vi "PickingControl.vi"(10 "PickingNumber":string, 11 "Machine":string) -> (0 "error out":errorcluster, 1 "Result":string, 2 "StatusURL":string, 3 "controlURL":string, 4 "DupResult":string)   [LabVIEW 2020]
uses:
  <vilib>/Utility/config.llb/Read Key (String).vi
  <vilib>/Utility/config.llb/NI_LVConfig.lvlib
panel:
  out "Status":bool
  in  "STOP":bool
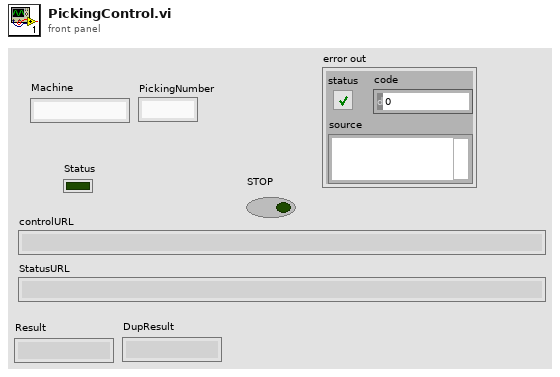
[diagram p1: front panel]
types:
  T1 = typedef "NI_LVConfig.lvlib/Config Data RefNum.ctl" = refnum<k1>
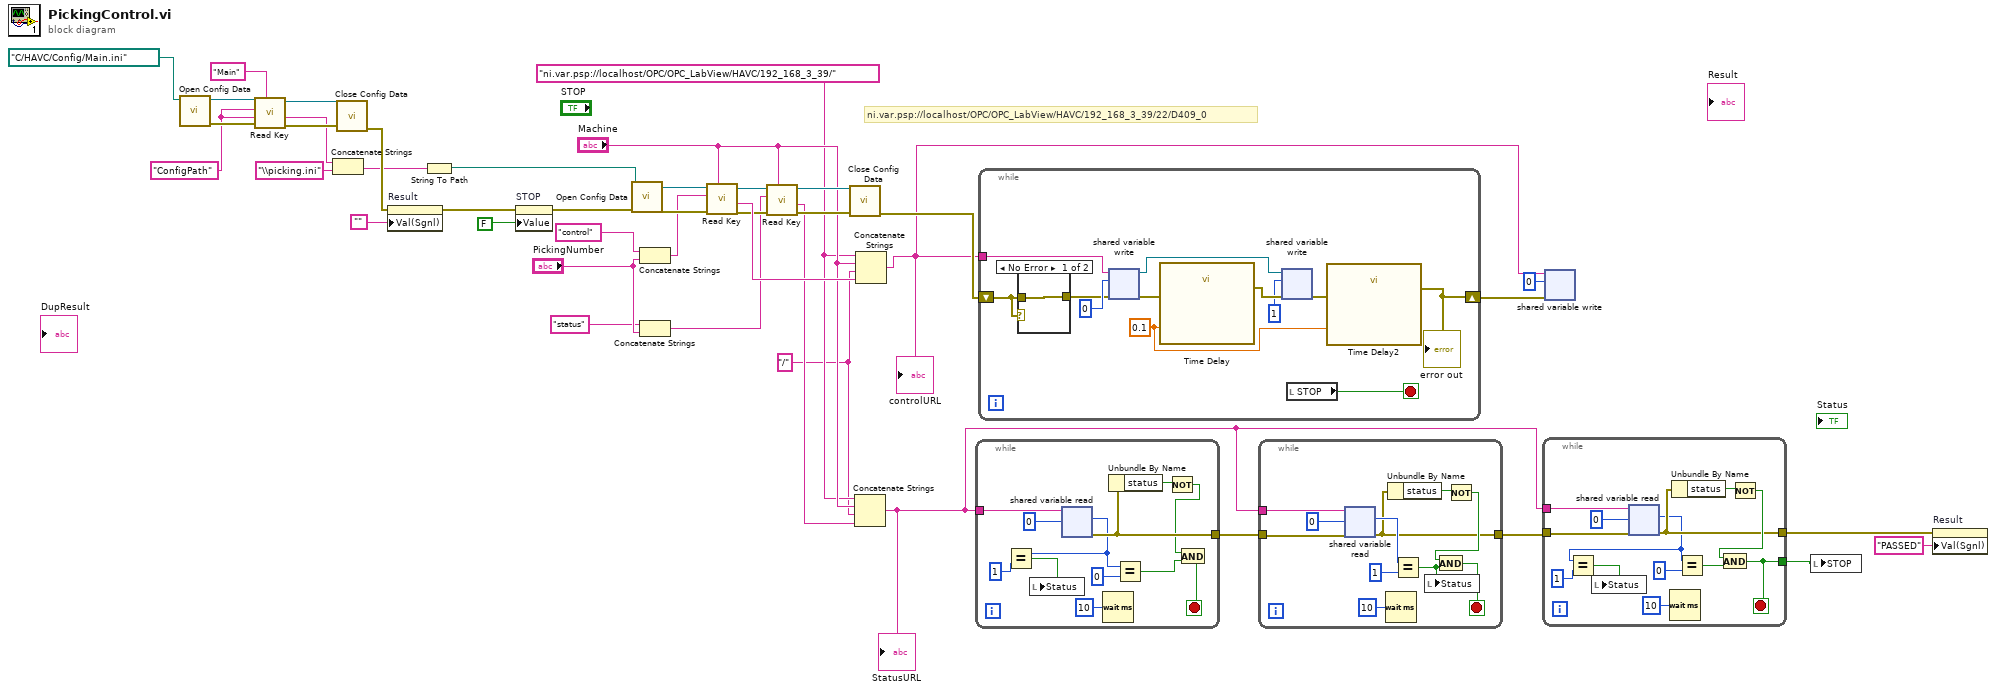
[diagram p0: block diagram]
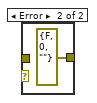
[diagram p2: hidden frame]
diagram:
  w5 = "ConfigPath" ("key")
  w22 = "/" ("string")
  w28 = "ni.var.psp://localhost/OPC/OPC_LabView/HAVC/192_168_3_39/" ("string")
  # "ni.var.psp://localhost/OPC/OPC_LabView/HAVC/192_168_3_39/22/D409_0"
  n1 = call <vilib>:"Open Config Data.vi"("configuration file path"=path "C:/HAVC/Config/Main.ini") -> ("error out"=w11:errorcluster, "refnum"=w10:T1)  [unwired: 8 in, 1 out]
  n2 = call-poly <vilib>:"Read Key.vi"("section"="Main", "error in (no error)"=w11, "default value"=w5, "key"=w5, "refnum"=w10) -> ("error out"=w8:errorcluster, "value"=w4:string, "refnum out"=w9:T1)  [unwired: 3 in, 1 out]
  n3 = Concatenate Strings(w4, "\\picking.ini" ("string")) -> (w2:string)
  n4 = call <vilib>:"Close Config Data.vi"("error in (no error)"=w8, "refnum"=w9) -> ("error out"=w7:errorcluster)  [unwired: 8 in, 1 out]
  n5 = property on="Result" class="Str"(error in=w7, "Val(Sgnl)"="") -> (error out=w14:errorcluster)  [unwired: 1 in, 1 out]
  n6 = String To Path(string=w2) -> (path=w1:path)
  n7 = property on="STOP" class="Bool (strict)"(error in=w14, "Value"=FALSE ("STOP")) -> (error out=w20:errorcluster)  [unwired: 1 in, 1 out]
  n8 = call <vilib>:"Open Config Data.vi"("error in (no error)"=w20, "configuration file path"=w1) -> ("error out"=w42:errorcluster, "refnum"=w41:T1)  [unwired: 7 in, 1 out]
  n9 = Concatenate Strings("control", "PickingNumber") -> (w39:string)
  n10 = Concatenate Strings("status" ("string"), "PickingNumber") -> (w30:string)
  n11 = call-poly <vilib>:"Read Key.vi"("section"="Machine", "error in (no error)"=w42, "key"=w39, "refnum"=w41) -> ("error out"=w34:errorcluster, "value"=w38:string, "refnum out"=w33:T1)  [unwired: 4 in, 1 out]
  n12 = call-poly <vilib>:"Read Key.vi"("section"="Machine", "error in (no error)"=w34, "key"=w30, "refnum"=w33) -> ("error out"=w31:errorcluster, "value"=w23:string, "refnum out"=w32:T1)  [unwired: 4 in, 1 out]
  n13 = call <vilib>:"Close Config Data.vi"("error in (no error)"=w31, "refnum"=w32) -> ("error out"=w37:errorcluster)  [unwired: 8 in, 1 out]
  n14 = Concatenate Strings(w28, "Machine", w22, w23) -> (w25:string)
  "StatusURL" <- w25
  n15 = Concatenate Strings(w28, "Machine", w22, w38) -> (w18:string)
  "controlURL" <- w18
  n16 = while {
    tunnel: w25 -> [w53]
    tunnel: [w49] -> w27
    stop <- w50 stop-if-true
    n17 = shared-variable-read(w53, 0) -> (w49:errorcluster, w45:i32)  [unwired: 1 in, 2 out]
    n18 = Equal?(x=w45, y=1) -> (x = y?=w43:bool)
    n19 = local write "Status"(w43) -> ()
    n20 = Wait (ms)(milliseconds to wait=u32 10) -> ()  [unwired: 1 out]
    n21 = Unbundle By Name(w49) -> ("status"=w48:bool)
    n22 = Equal?(x=w45, y=0) -> (x = y?=w46:bool)
    n23 = Not(x=w48) -> (.not. x?=w47:bool)
    n24 = And(x=w47, y=w46) -> (x .and. y?=w50:bool)
  }
  n25 = while {
    shift-right: [w57] -> w19
    shift-left: w37 -> [w61]
    tunnel: w18 -> [w59]
    stop <- w55 stop-if-true
    w56 = 0.1 ("Delay Time (s)")
    n26 = case shown="No Error" w61 {
      tunnel: w61 -> [w67 _]
      tunnel: [w67 errorcluster {"status"=FALSE, "code"=0, "source"=""} ("error IO")] -> w60
      frame No Error {
      }
      frame Error {
      }
    }
    n27 = shared-variable-write(w59, w60, 0) -> (w65:refnum<k21>, w66:errorcluster)
    n28 = call "Time Delay"("error in (no error)"=w66, "Delay Time (s)"=w56) -> ("error out"=w64:errorcluster)  [unwired: 9 in]
    n29 = shared-variable-write(w65, w64, 1) -> (w58:errorcluster)  [unwired: 1 out]
    n30 = local read "STOP"() -> (w55:bool)
    n31 = call "Time Delay2"("error in (no error)"=w58, "Delay Time (s)"=w56) -> ("error out"=w57:errorcluster)  [unwired: 9 in]
    "error out" <- w57
  }
  n32 = while {
    tunnel: w25 -> [w78]
    tunnel: w27 -> [w74]
    tunnel: [w70] -> w26
    stop <- w72 stop-if-true
    n33 = shared-variable-read(w78, w74, 0) -> (w70:errorcluster, w76:i32)  [unwired: 2 out]
    n34 = Wait (ms)(milliseconds to wait=u32 10) -> ()  [unwired: 1 out]
    n35 = Unbundle By Name(w70) -> ("status"=w73:bool)
    n36 = Equal?(x=w76, y=1) -> (x = y?=w69:bool)
    n37 = local write "Status"(w69) -> ()
    n38 = Not(x=w73) -> (.not. x?=w71:bool)
    n39 = And(x=w71, y=w69) -> (x .and. y?=w72:bool)
  }
  n40 = while {
    tunnel: w25 -> [w91]
    tunnel: w26 -> [w88]
    tunnel: [w85] -> w16
    tunnel: [w84] -> w24
    stop <- w84 stop-if-true
    n41 = shared-variable-read(w91, w88, 0) -> (w85:errorcluster, w81:i32)  [unwired: 2 out]
    n42 = Equal?(x=w81, y=1) -> (x = y?=w80:bool)
    n43 = local write "Status"(w80) -> ()
    n44 = Wait (ms)(milliseconds to wait=u32 10) -> ()  [unwired: 1 out]
    n45 = Unbundle By Name(w85) -> ("status"=w87:bool)
    n46 = Equal?(x=w81, y=0) -> (x = y?=w83:bool)
    n47 = Not(x=w87) -> (.not. x?=w86:bool)
    n48 = And(x=w86, y=w83) -> (x .and. y?=w84:bool)
  }
  n49 = shared-variable-write(w18, w19, 0 ("data in")) -> ()  [unwired: 2 out]
  n50 = local write "STOP"(w24) -> ()
  n51 = property on="Result" class="Str"(error in=w16, "Val(Sgnl)"="PASSED" ("Value (Signaling)")) -> ()  [unwired: 1 in, 2 out]
